vi "JoystickToggleCounter.vi"(1 "Button":bool, 2 "Number of positions":i8) -> (0 "Counter":i32)   [LabVIEW 2011]
panel:
  in  "Numeric":i8
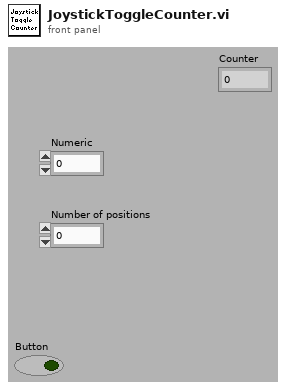
[diagram p1: front panel]
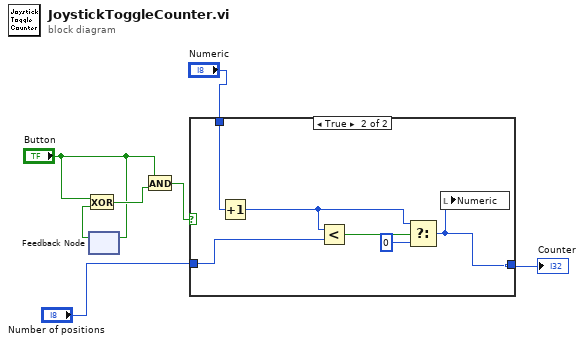
[diagram p0: block diagram]
diagram:
  n1 = feedback-in #1("Button") -> ()
  n2 = feedback #1() -> (w2:bool)  [unwired: 1 out]
  n3 = Exclusive Or(1:w2, 2:"Button") -> (0:w5:bool)
  n4 = And(x="Button", y=w5) -> (x .and. y?=w4:bool)
  n5 = case shown="True" w4 {
    tunnel: [w8 w9] -> w6
    tunnel: "Number of positions" -> [_ w11]
    tunnel: "Numeric" -> [w8 w10]
    frame False {
    }
    frame True {
      n6 = Increment(x=w10) -> (x+1=w13:i8)
      n7 = Less?(x=w13, y=w11) -> (x < y?=w14:bool)
      n8 = Select(t=w13, s=w14, f=0) -> (s? t:f=w9:i32)
      n9 = local write "Numeric"(w9) -> ()
    }
  }
  "Counter" <- w6
